vi "setBoardID.vi"(8 "error in (no error)":errorcluster, 10 "boardID":i32, 11 "Pixelfly in":refnum<class "Pixelfly.lvclass">) -> (0 "error out":errorcluster, 3 "Pixelfly out":refnum<class "Pixelfly.lvclass">)   [LabVIEW 2009, in "Hardware.lvlib" / "Channels.lvlib" / "Pixelfly.lvclass"]
uses:
  Pixelfly.lvclass
  Pixelfly.lvclass/Pixelfly.ctl
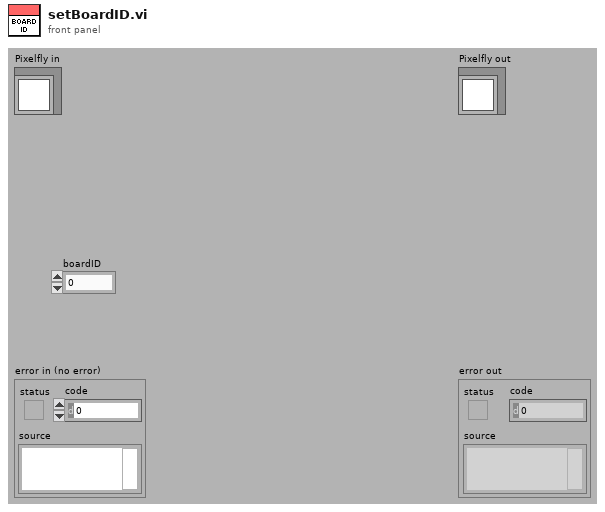
[diagram p1: front panel]
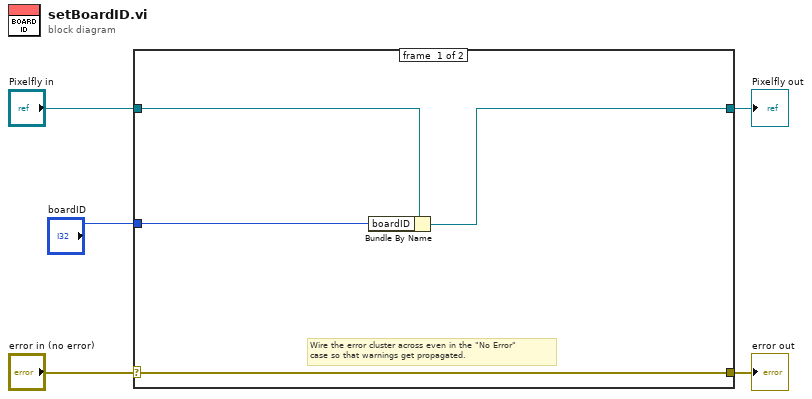
[diagram p0: block diagram]
diagram:
  n1 = case shown="No Error" "error in (no error)" {
    selector: "error in (no error)" -> [w9 w11]
    tunnel: [w9 w11] -> w4
    tunnel: [w6 w10] -> w2
    tunnel: "Pixelfly in" -> [w7 w10]
    tunnel: "boardID" -> [w8 _]
    frame #0 {
      # "Wire the error cluster across even in the \"No Error\"\ncase so that warnings get propagated."
      n2 = Bundle By Name(cluster=w7, "boardID"=w8) -> (w6:refnum<class "Pixelfly.lvclass">)
    }
    frame #1 {
    }
  }
  "error out" <- w4
  "Pixelfly out" <- w2
